vi "Read Humidity (%).vi"(8 "error in (no error)":errorcluster, 11 "HTS221 in":refnum<class "HTS221.lvclass">) -> (0 "error out":errorcluster, 2 "Relative Humidity (%)":dbl, 3 "HTS221 out":refnum<class "HTS221.lvclass">)   [LabVIEW 2020, in "HTS221.lvclass"]
uses:
  HTS221.lvclass
  HTS221.lvclass/HTS221.ctl
  Read Humidity.Zero.vi
  Read Humidity.Slope.vi
  LINX I2C/LINX I2C.lvclass
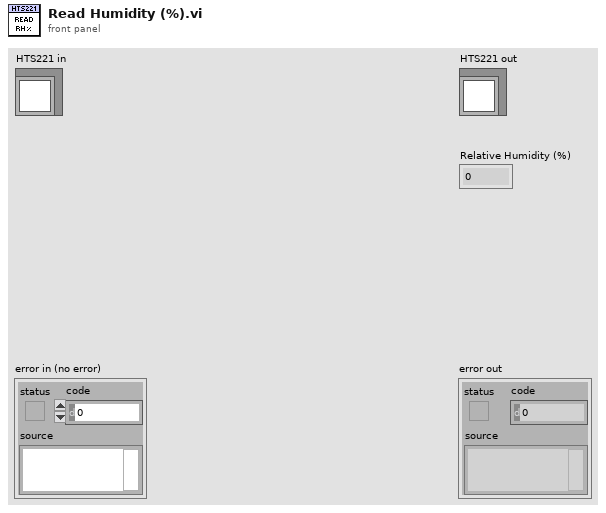
[diagram p1: front panel]
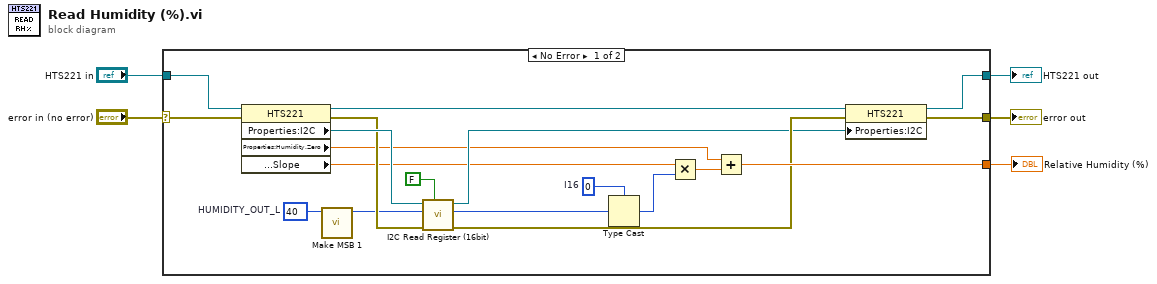
[diagram p0: block diagram]
diagram:
  n1 = case shown="No Error" "error in (no error)" {
    selector: "error in (no error)" -> [w23 w26]
    tunnel: [w13 w26] -> w4
    tunnel: [w15 w25] -> w2
    tunnel: "HTS221 in" -> [w24 w25]
    tunnel: [w22 _] -> w1
    frame No Error {
      w9 = u8 40  # HUMIDITY_OUT_L
      w19 = i16 0  # I16
      n2 = property class="HTS221"(reference=w24, error in=w23) -> (reference out=w16:refnum<class "HTS221.lvclass">, error out=w20:errorcluster, "Properties:I2C"=w21:refnum<class "LINX I2C.lvclass">, "Properties:Humidity.Zero"=w11:dbl, "Properties:Humidity.Slope"=w12:dbl)
      n3 = call "Make MSB 1.vi"("Register Address"=w9) -> ("Register Address | 0x80"=w8:u8)  [unwired: 10 in]
      n4 = call "I2C Read Register (16bit).vi"("MSB(yte) First? (F=Lo->Hi)"=FALSE ("MSB(yte) First? (T)"), "error in (no error)"=w20, "Register Address"=w8, "LINX I2C in"=w21) -> ("error out"=w17:errorcluster, "Value"=w7:u16, "LINX I2C out"=w14:refnum<class "LINX I2C.lvclass">)  [unwired: 5 in]
      n5 = Type Cast(type=w19, x=w7) -> (*(type *) &x=w18:i16)
      n6 = Multiply(x=w12, y=w18) -> (x*y=w10:dbl)
      n7 = Add(x=w11, y=w10) -> (x+y=w22:dbl)
      n8 = property class="HTS221"(reference=w16, error in=w17, "Properties:I2C"=w14) -> (reference out=w15:refnum<class "HTS221.lvclass">, error out=w13:errorcluster)
    }
    frame Error {
    }
  }
  "error out" <- w4
  "HTS221 out" <- w2
  "Relative Humidity (%)" <- w1
